vi "setArmStimulus.vi"(8 "error in (no error)":errorcluster, 10 "channel":i32, 11 "K2602 in":refnum<class "K2602.lvclass">) -> (0 "error out":errorcluster, 3 "K2602 out":refnum<class "K2602.lvclass">)   [LabVIEW 2011, in "Hardware.lvlib" / "Channels.lvlib" / "K2602.lvclass"]
uses:
  K2602.lvclass
  K2602.lvclass/K2602.ctl
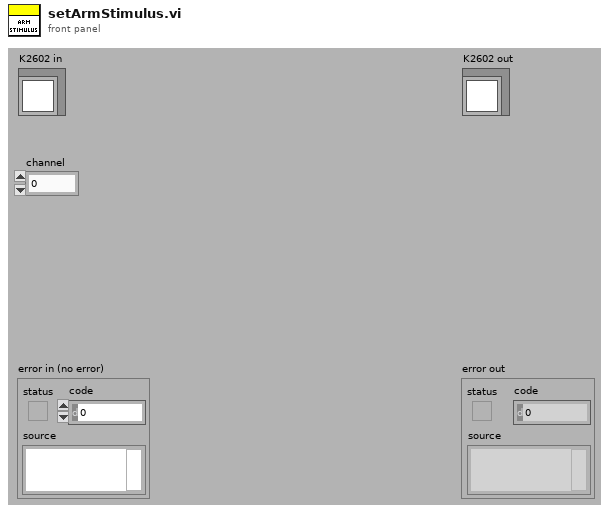
[diagram p1: front panel]
types:
  T1 = cluster{"Range":cluster{"current":dbl, "voltage":dbl}, "triggering_inUse":cluster{"start_trigger":string, "clock":string}, "Limits":cluster{"VoltageLimit":dbl, "CurrentLimit":dbl}}[]
  T2 = cluster{"Range":cluster{"current":dbl, "voltage":dbl}, "triggering_inUse":cluster{"start_trigger":string, "clock":string}, "Limits":cluster{"VoltageLimit":dbl, "CurrentLimit":dbl}}
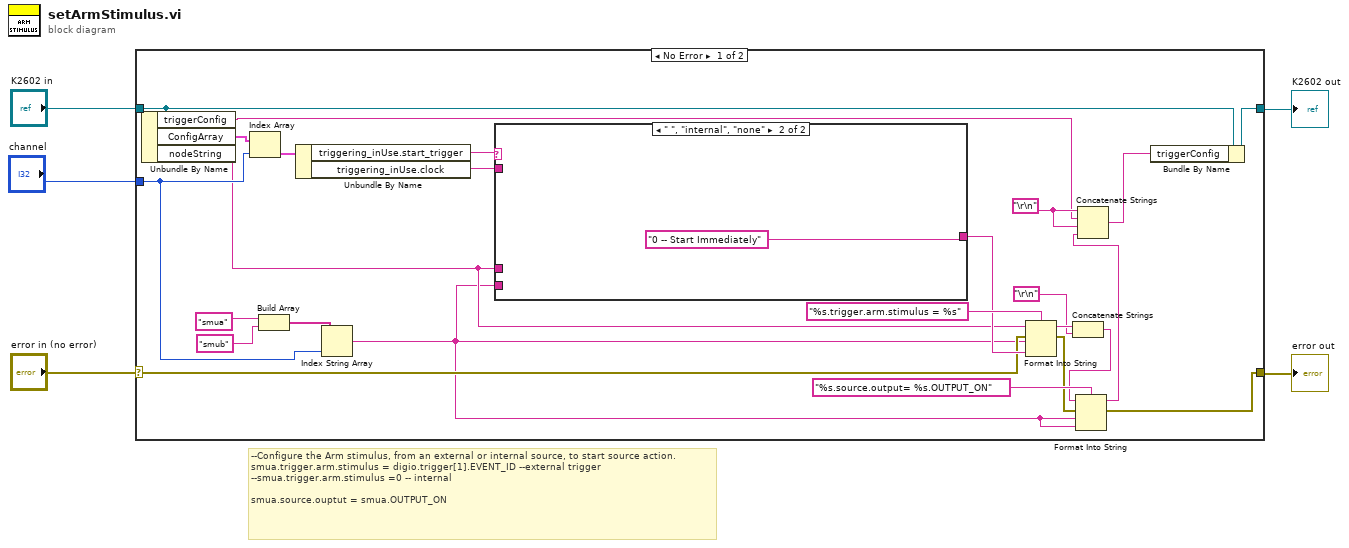
[diagram p0: block diagram]
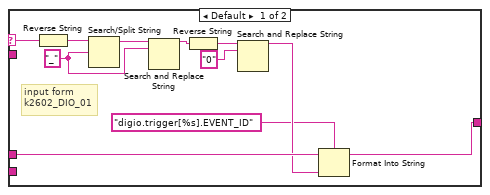
[diagram p2: hidden frame]
diagram:
  # "--Configure the Arm stimulus, from an external or internal source, to start source action.\nsmua.trigger.arm.stimulus = digio.trigger[1].EVENT_ID --external trigger\n--smua.trigger.arm.stimulus =0 -- internal \n\nsmua.source.ouptut = smua.OUTPUT_ON"
  n1 = case shown="No Error" "error in (no error)" {
    selector: "error in (no error)" -> [w20 w44]
    tunnel: [w11 w44] -> w4
    tunnel: [w14 w43] -> w2
    tunnel: "K2602 in" -> [w16 w43]
    tunnel: "channel" -> [w23 _]
    frame No Error {
      w18 = "\r\n"
      n2 = Unbundle By Name(w16) -> ("triggerConfig"=w17:string, "ConfigArray"=w30:T1, "nodeString"=w19:string)
      n3 = Index Array(array=w30, index=w23) -> (element=w29:T2)
      n4 = Build Array("smua", "smub") -> (w24:string[])
      n5 = Unbundle By Name(w29) -> ("triggering_inUse.start_trigger"=w28:string, "triggering_inUse.clock"=w27:string)
      n6 = Index String Array(1:w23, 2:w24) -> (0:w10:string)  [unwired: 1 in]
      n7 = case shown="\" \", \"internal\", \"none\"" w28 {
        selector: w28 -> [w41 _]
        tunnel: w27 -> [_ _]
        tunnel: w19 -> [w34 _]
        tunnel: [w31 "0 -- Start Immediately"] -> w21
        tunnel: w10 -> [_ _]
        frame Default {
          w38 = "_"
          # "input form\nk2602_DIO_01"
          n8 = Reverse String(1:w41) -> (0:w40:string)
          n9 = Search/Split String(string=w40, search string/char (-)=w38) -> (substring before match=w39:string)  [unwired: 1 in, 2 out]
          n10 = Search and Replace String(input string=w39, search string=w38) -> (result string=w37:string)  [unwired: 6 in, 3 out]
          n11 = Reverse String(1:w37) -> (0:w36:string)
          n12 = Search and Replace String(input string=w36, search string="0") -> (result string=w33:string)  [unwired: 6 in, 3 out]
          n13 = Format Into String(format string="digio.trigger[%s].EVENT_ID", initial string=w34, w33) -> (resulting string=w31:string)  [unwired: 1 in, 1 out]
        }
        frame " ", "internal", "none" {
        }
      }
      n14 = Format Into String(format string="%s.trigger.arm.stimulus = %s", initial string=w19, error in=w20, w10, w21) -> (resulting string=w8:string, error out=w12:errorcluster)
      n15 = Concatenate Strings(w8, "\r\n") -> (w6:string)
      n16 = Format Into String(format string="%s.source.output= %s.OUTPUT_ON", initial string=w6, error in=w12, w10, w10) -> (resulting string=w9:string, error out=w11:errorcluster)
      n17 = Concatenate Strings(w18, w17, w18, w9) -> (w15:string)
      n18 = Bundle By Name(cluster=w16, "triggerConfig"=w15) -> (w14:refnum<class "K2602.lvclass">)
    }
    frame Error {
    }
  }
  "error out" <- w4
  "K2602 out" <- w2
